vi "Gestion Erreur.vi"(8 "error in (no error)":errorcluster caption="entrée d'erreur (pas d'erreur)", 11 "Sequenceur ?":bool) -> (0 "error out":errorcluster caption="sortie d'erreur")   [LabVIEW 2020]
uses:
  TypeDef/Liste Fonction appelante.ctl
  TypeDef/Liste Event Sequenceur.ctl
  TypeDef/Data Event Sequenceur.ctl
  IHM/Variable globale.vi
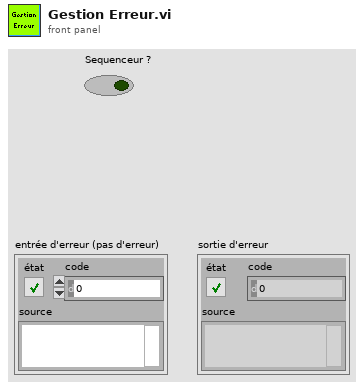
[diagram p1: front panel]
types:
  T1 = typedef "Liste Fonction appelante.ctl" = enum16{"None", "Open Com DUT", "Enter OF", "Serial Number", "Start-up", "Start Test", "Finish", "Enter S/N PWR", "Enter S/N ANT", "Read Mac Address", "Test Frequency", "Initialization", "ID EnOcean", "ID Wirepass", "Test Button", "Test EEPROM", "Test LED", "Test Relay", "Test RTC", "Reset Factory", "Read parameter", "Programm Software", "Programm FW", "IHM", "Print Label PCBA", "Print Label Assembled", "Print Label Packaging", "End", "Error"}
  T2 = typedef "Liste Event Sequenceur.ctl" = enum16{"None", "------Commun------", "Quit", "Stop", "Next Test ", "Increment state", "Command VBat", "Command 5V", "Command 24V", "Command Tension 1", "Command Tension 2", "Command Tension 3", "Stop Power Supply", "Wait Power Supply", "Msg Start-up", "Start Test", "--------Test---------", "Finish", "Enter S/N PWR", "Enter S/N ANT", "Initialization", "ID EnOcean", "ID Wirepass", "ID Wirepass By J-link", "Read Mac Address", "Test EEPROM", "Programm Software", "Programm FW", "Test LED", "Test Relay", "Test RTC", "Test Button", "Reset Factory", "Test Frequency", "Read parameter", "-------Fonction-------", "Get Manufacturer ID", "Write Key", "Read Key", "Write UID", "Read UID", "Factory Reset", "Activate Service BLE", "Factory Reset With Return", "Get device type", "Teach-In EnOcean", "Get Link Table", "Get product ID", "Learn In", "Read ID EnOcean", "Read ID Wirepass", "Read ID Wirepass By J-link", "Calibration Frequency", "Get FW version", "Get HW version", "Set HW version ANT", "Set HW version PWR", "Set S/N & HW Version", "Get Serial number", "Get mode", "Set Mode Scheduler", "Set Mode Zigbee", "Get BLE Address", "Get ZB Address", "Get RTC", "Set RTC", "Get Relay status", "Set Relay On Ch1", "Set Relay Off Ch1", "Set Relay On Ch2", "Set Relay Off Ch2", "LED Red", "LED Orange", "LED Green", "LED Off", "Read Status Button", "Read Status Switch 1", "Read Status Switch 2", "Init Ok", "-------Fonction de base-----", "Programm With J-link", "Erase All with NRF Tools", "Programm Bootloader With Commander", "Programm Erase With Commander", "Programm Applicatif With Commander", "Programm Test With Commander", "Calibration Frequency With Commander", "Init Calibration Frequency With Commander", "Encode S/N", "Creation S/N", "Save S/N", "Reset S/N", "Programm DFU", "Erase CPU", "Enable Jlink", "Disable Jlink", "Enable ICD", "Disable ICD", "Enable UART", "Disable UART", "Enable Alim Produit", "Disable Alim Produit", "Enable SW1", "Disable SW1", "Enable SW2", "Disable SW2", "Enable Multi 220V", "Disable Multi 220V", "Enable Multi V1", "Enable Multi V2", "Enable Multi V3", "Enable Multi V4", "Enable Multi V5", "Enable Multi V6", "Enable Multi V7", "Enable Multi V8", "Disable Multi", "Enable EV1", "Enable EV2", "Enable EV3", "Enable CS1", "Enable CS2", "Enable CS3", "Enable CS4", "Disable DO", "Wait Frequency", "Wait Press", "Wait Event Press", "Wait Release", "Wait Event Release", "Wait turn", "Wait Move", "Wait Remove", "Wait Power", "Waiting Back BLE", "Connect BLE", "Disconnect BLE", "Waiting Back RS", "Waiting Back SSH", "Waiting Display Operator", "Operator Input", "Operator Waiting Show", "Operator Waiting mask", "Waiting Operator", "Waiting Operator Input", "BLE Read RSSI", "Read DIO", "Read Ana 1", "Read Ana 2", "Read Ana 3", "Read Ana 4", "Read Ana 5", "Read Ana 6", "Read Ana 7", "Read Ana 8", "Write Ana 1", "Write Ana 2", "Ammeter Reading DC", "Ammeter Reading AC", "Multimeter Reading DC", "Multimeter Reading AC", "LED FEASA Reading", "Tempo 1", "Tempo 2", "Tempo 3", "Tempo 4", "Tempo 5", "Tempo 6", "Sanction", "No Sanction", "Print Label", "Write CSV", "Send Mail"}
  T3 = typedef "Data Event Sequenceur.ctl" = cluster{"Data":variant, "Action":T2, "Fonction Appelante":T1, "TimeOut ou Tempo":u32, "Nb Répétition":i32, "Nom étape":string}
  T4 = typedef "File et notification.ctl" = cluster{"Arret Appli":refnum<notifier>, "Erreur Acqui":refnum<notifier>, "File Event Sequenceur":refnum<queue>, "Liste test à faire":refnum<queue>, "File Event Historique":refnum<queue>, "Variable Global":refnum<notifier>, "Variable stocke retour Etat":refnum<notifier>, "Retour Validation OP":refnum<queue>, "Demande Validation OP":refnum<queue>, "Retour Autotest":refnum<notifier>, "Demande Autotest":refnum<queue>, "Adr Mac Produit":refnum<notifier>, "Autorise commande":refnum<notifier>, "Event Init BLE":refnum<notifier>, "Action Lecture RS":refnum<queue>, "Key produit":refnum<notifier>, "Retour Saisie OP":refnum<queue>, "Demande Saisie OP":refnum<queue>, "Etat flashage":refnum<notifier>, "Code Operateur":refnum<notifier>, "Resultat test Global":refnum<notifier>, "Stop Test":refnum<notifier>, "Init IHM Autotest":refnum<notifier>, "Version test bench":refnum<notifier>, "SN Product":refnum<notifier>, "En erreur":refnum<notifier>, "Affiche Result":refnum<queue>, "S/N PWR":refnum<notifier>, "AppEUI":refnum<notifier>, "Action Lecture Temp":refnum<queue>, "Temp":refnum<notifier>, "AppKey":refnum<notifier>, "OF":refnum<notifier>, "File Commande Shielding":refnum<queue>, "Return Status":refnum<notifier>, "ID Product":refnum<notifier>, "Version FW":refnum<notifier>, "Version HW":refnum<notifier>, "Adresse IHM":refnum<notifier>, "RTC":refnum<notifier>, "S/N Ant":refnum<notifier>, "SN Encode":refnum<notifier>, "Key Product":refnum<notifier>}
  T5 = typedef "Adresse IHM.ctl" = cluster{"TabGestionScénario":refnum<vi>, "MAJ TabTest":refnum<vi>, "MAJ IHM":refnum<vi>, "BpStop":refnum<vi>, "Autotest OK":refnum<vi>, "BpContinue":refnum<vi>, "BpStart":refnum<vi>, "Action en chinois":refnum<vi>, "Bouton vide":refnum<vi>, "StatusPCB":refnum<vi>, "StatusAssembled":refnum<vi>, "Bouton Exit":refnum<vi>, "Action En cours":refnum<vi>}
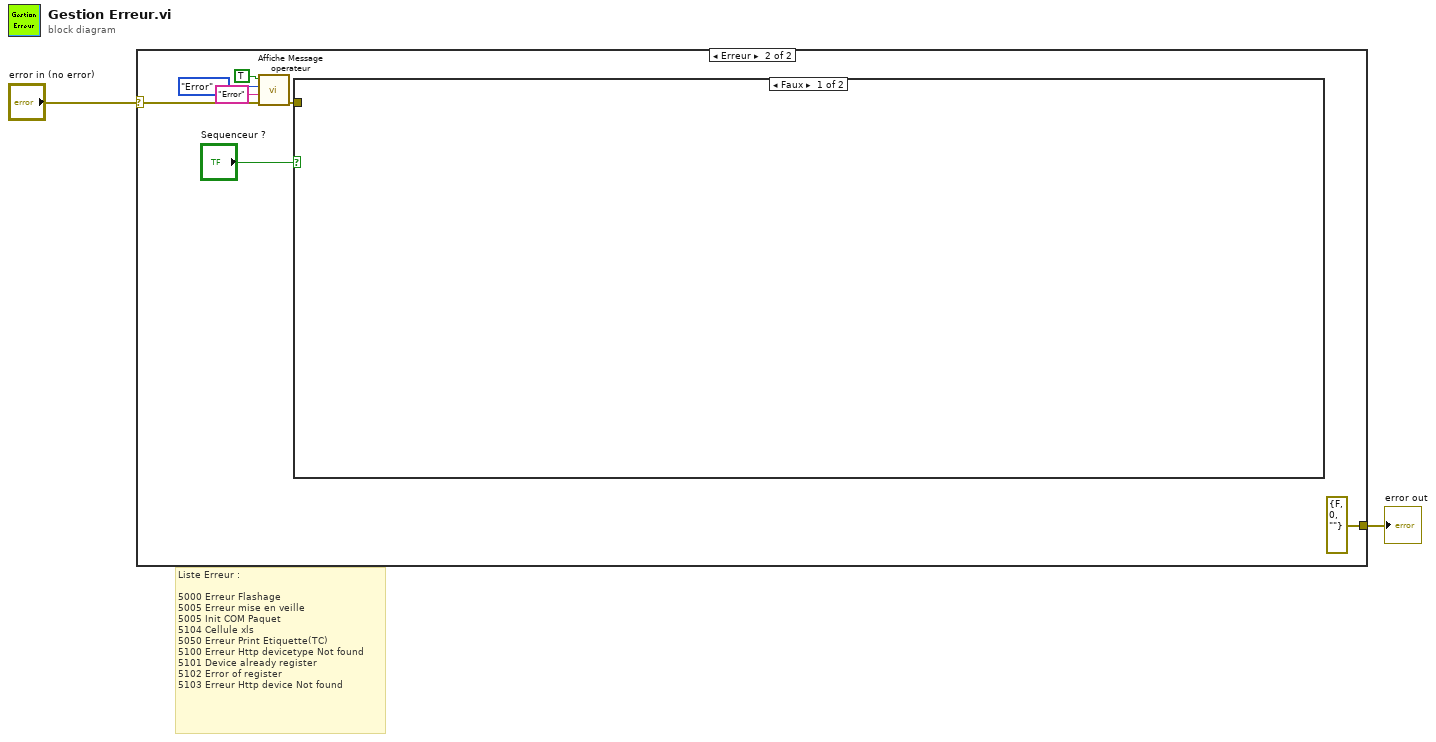
[diagram p0: block diagram]
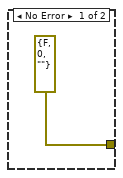
[diagram p2: hidden frame]
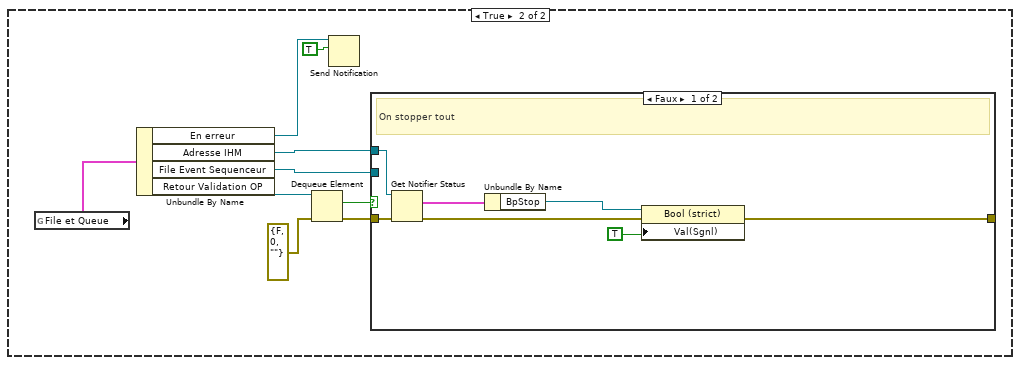
[diagram p3: hidden frame]
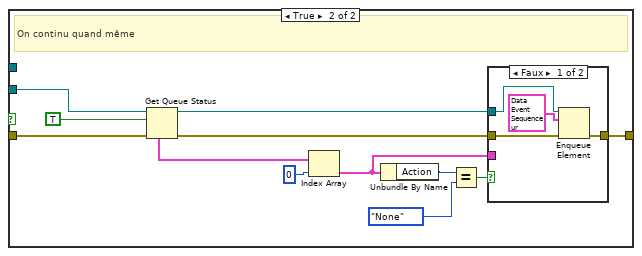
[diagram p4: hidden frame]
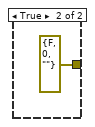
[diagram p5: hidden frame]
diagram:
  # "Liste Erreur :\n\n5000 Erreur Flashage\n5005 Erreur mise en veille\n5005 Init COM Paquet\n5104 Cellule xls \n5050 Erreur Print Etiquette(TC)\n5100 Erreur Http devicetype Not found \n5101 Device already register\n5102 Error of register\n5103 Erreur Http device Not found"
  n1 = case shown="Erreur" "error in (no error)" {
    selector: "error in (no error)" -> [_ w10]
    tunnel: [errorcluster {"status"=FALSE, "code"=0, "source"=""} ("error out") errorcluster {"status"=FALSE, "code"=0, "source"=""} ("error out")] -> w2
    frame No Error {
    }
    frame Error {
      n2 = call "Affiche Message operateur.vi"("error in (no error)"=w10, "Etat en cours"="Error", "Fonction Appelante"=Liste_Fonction_appelante."Error", "Afficher ?"=TRUE) -> ("error out"=w6:errorcluster)  [unwired: 7 in]
      n3 = case shown="Faux" "Sequenceur ?" {
        tunnel: w6 -> [_ _]
        frame False {
        }
        frame True {
          n4 = global read "Variable globale.vi" "File et Queue"() -> (w11:T4)
          n5 = Unbundle By Name(w11) -> ("En erreur"=w12:refnum<notifier>, "Adresse IHM"=w14:refnum<notifier>, "File Event Sequenceur"=w16:refnum<queue>, "Retour Validation OP"=w18:refnum<queue>)
          n6 = Dequeue Element(queue=w18, error in (no error)=errorcluster {"status"=FALSE, "code"=0, "source"=""} ("error out")) -> (element=w15:bool, error out=w17:errorcluster)  [unwired: 1 in, 2 out]
          n7 = Send Notification(notification=TRUE, notifier=w12) -> ()  [unwired: 1 in, 2 out]
          n8 = case shown="Faux" w15 {
            tunnel: w17 -> [w24 w38]
            tunnel: w16 -> [_ w37]
            tunnel: [w25 w28] -> _
            tunnel: w14 -> [w23 _]
            frame False {
              # "On stopper tout"
              n9 = Get Notifier Status(notifier=w23, error in (no error)=w24) -> (current notification=w22:T5, error out=w20:errorcluster)  [unwired: 3 out]
              n10 = Unbundle By Name(w22) -> ("BpStop"=w21:refnum<vi>)
              n11 = property class="Bool (strict)"(reference=w21, error in=w20, "Val(Sgnl)"=TRUE) -> (error out=w25:errorcluster)  [unwired: 1 out]
            }
            frame True {
              # "On continu quand même"
              n12 = Get Queue Status(queue=w37, return elements? (F)=TRUE ("renvoyer les éléments ? (F)"), error in (no error)=w38) -> (queue out=w27:refnum<queue>, error out=w30:errorcluster, elements=w34:T3[])  [unwired: 5 out]
              n13 = Index Array(array=w34, index=0 ("indice")) -> (element=w29:T3)
              n14 = Unbundle By Name(w29) -> ("Action"=w35:T2)
              n15 = Equal?(x=w35, y=Liste_Event_Sequenceur."None") -> (x = y?=w31:bool)
              n16 = case shown="Faux" w31 {
                tunnel: w30 -> [w41 _]
                tunnel: w29 -> [_ _]
                tunnel: [w40 errorcluster {"status"=FALSE, "code"=0, "source"=""} ("error out")] -> w28
                tunnel: w27 -> [w39 _]
                frame False {
                  n17 = Enqueue Element(queue=w39, element=T3 {"Data"=variant, "Action"=enum."None", "Fonction Appelante"=enum."None", "TimeOut ou Tempo"=0, "Nb Répétition"=0, "Nom étape"=""} ("cas faux"), error in (no error)=w41) -> (error out=w40:errorcluster)  [unwired: 1 in, 2 out]
                }
                frame True {
                }
              }
            }
          }
        }
      }
    }
  }
  "error out" <- w2
